vi "cm2nm_find_pairs_of_fiducials.vi"(3 "CurrentSessionFiducialLocations":cluster{"X":dbl, "Y":dbl, "Z":dbl}[](array[cluster]), 4 "ReferenceFiducialLocations":cluster{"X":dbl, "Y":dbl, "Z":dbl}[](array[cluster])) -> (0 "IndexRefrenceSession":i32[](array[numeric]), 1 "min_distance":dbl, 2 "IndexCurrentSession":i32[](array[numeric]))   [LabVIEW 2011]
doc: "from two sessions resolve the pairing of the fiducials from the location. assumes the session with the least number of fiducials is a subset of the equal or larger set of fiducials."
panel:
  in  "index":i32
  in  "stop":bool
  out "XY Graph":cluster{dbl[], dbl[]}[](graph)
  out "Waveform Graph":dbl[](graph)
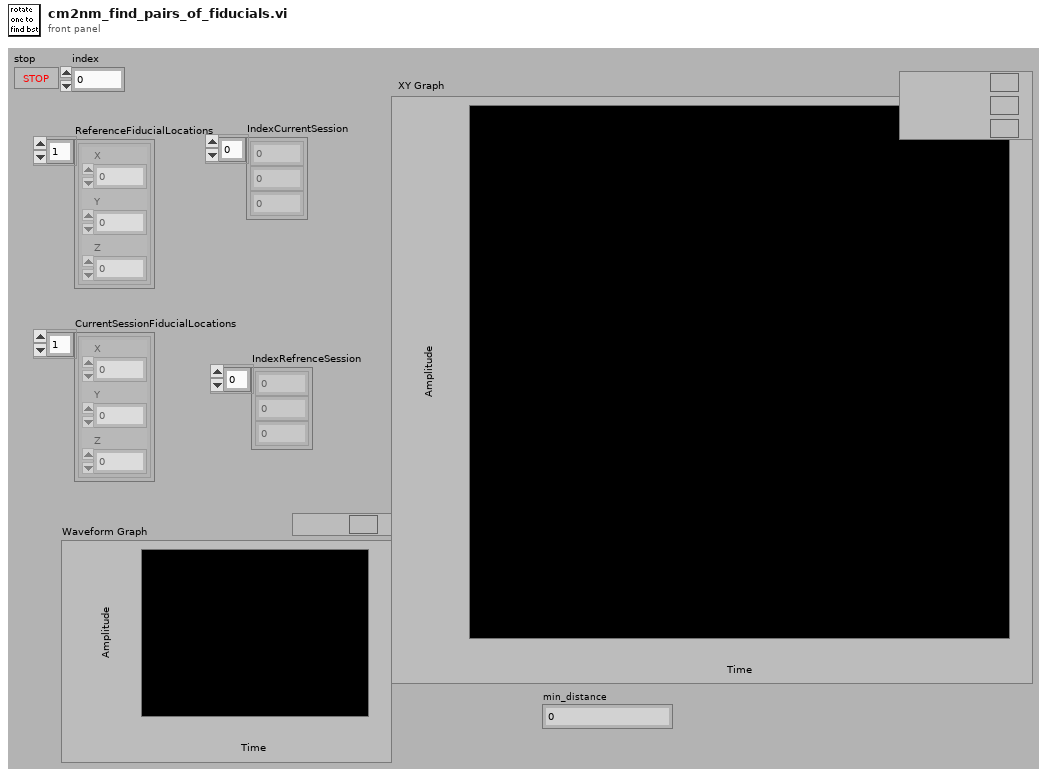
[diagram p1: front panel]
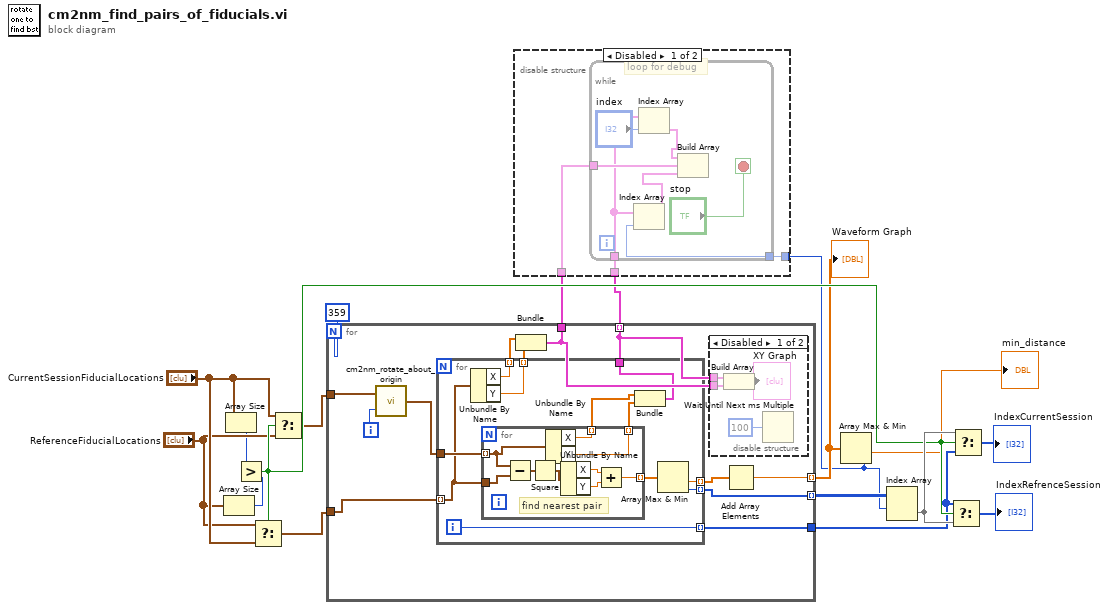
[diagram p0: block diagram]
diagram:
  n1 = Array Size(array="ReferenceFiducialLocations") -> (size(s)=w8:i32)
  n2 = Array Size(array="CurrentSessionFiducialLocations") -> (size(s)=w7:i32)
  n3 = Greater?(x=w7, y=w8) -> (0:w14:bool)
  n4 = Select(t="ReferenceFiducialLocations", s=w14, f="CurrentSessionFiducialLocations") -> (s? t:f=w13:cluster{"X":dbl, "Y":dbl, "Z":dbl}[])
  n5 = Select(t="CurrentSessionFiducialLocations", s=w14, f="ReferenceFiducialLocations") -> (s? t:f=w11:cluster{"X":dbl, "Y":dbl, "Z":dbl}[])
  n6 = for {
    N: 359 -> [_]
    tunnel: w11 -> [w30]
    tunnel: w13 -> [w24]
    tunnel: [w28] -> w10 mode=indexing
    tunnel: [w27] -> w9 mode=indexing
    tunnel: [w26] -> w5
    tunnel: [w19] -> w4
    tunnel: [w20] -> w3 mode=indexing
    i -> [w23]
    n7 = call "cm2nm_rotate_about_origin.vi"("Theta(deg)"=w23, "In"=w30) -> ("Rotated"=w25:cluster{"X":dbl, "Y":dbl, "Z":dbl}[])
    n8 = for {
      tunnel: w24 -> [w40] mode=indexing
      tunnel: w25 -> [w45]
      tunnel: [w43] -> w29 mode=indexing
      tunnel: [w42] -> w28 mode=indexing
      tunnel: [w41] -> w26 mode=indexing
      tunnel: [w37] -> w20
      tunnel: [w36] -> w22 mode=indexing
      tunnel: [w35] -> w21 mode=indexing
      i -> [w41]
      n9 = Unbundle By Name(w40) -> ("X"=w36:dbl, "Y"=w35:dbl)
      n10 = for {
        tunnel: w45 -> [w49] mode=indexing
        tunnel: w40 -> [w54]
        tunnel: [w51] -> w44 mode=indexing
        tunnel: [w47] -> w39 mode=indexing
        tunnel: [w46] -> w38 mode=indexing
        # "find nearest pair"
        n11 = Subtract(x=w49, y=w54) -> (x-y=w50:cluster{"X":dbl, "Y":dbl, "Z":dbl})
        n12 = Square(x=w50) -> (x^2=w53:cluster{"X":dbl, "Y":dbl, "Z":dbl})
        n13 = Unbundle By Name(w49) -> ("X"=w47:dbl, "Y"=w46:dbl)
        n14 = Unbundle By Name(w53) -> ("X"=w48:dbl, "Y"=w52:dbl)
        n15 = Add(x=w48, y=w52) -> (x+y=w51:dbl)
      }
      n16 = Bundle(w39, w38) -> (w37:cluster{dbl[], dbl[]})  [unwired: 1 out]
      n17 = Array Max & Min(array=w44) -> (min value=w43:dbl, min index (indices)=w42:i32)  [unwired: 2 out]
    }
    n18 = Bundle(w22, w21) -> (w19:cluster{dbl[], dbl[]})  [unwired: 1 out]
    n19 = disable-structure shown="Disabled" {
      disable-tunnel: w20 -> [w34 _]
      disable-tunnel: w19 -> [w33 _]
      frame Disabled {
        n20 = Build Array(w34, w33) -> (→"XY Graph":cluster{dbl[], dbl[]}[])
        n21 = Wait Until Next ms Multiple(millisecond multiple=u32 100) -> ()  [unwired: 1 out]
      }
      frame Enabled {
      }
    }
    n22 = Add Array Elements(numeric array=w29) -> (sum=w27:dbl)
  }
  "Waveform Graph" <- w9
  n23 = Array Max & Min(array=w9) -> (min value=→"min_distance":dbl, min index (indices)=w2:i32)  [unwired: 2 out]
  n24 = disable-structure shown="Disabled" {
    disable-tunnel: w4 -> [w57 _]
    disable-tunnel: w3 -> [w56 _]
    disable-tunnel: w2 -> [w55 _]
    frame Disabled {
      # "loop for debug"
      n25 = while {
        tunnel: w57 -> [w65]
        tunnel: w56 -> [w60]
        tunnel: w55 -> [w63]
        stop <- "stop" stop-if-true
        n26 = Index Array(array=w60, index=w63) -> (element=w62:cluster{dbl[], dbl[]})
        n27 = Index Array(array=w60, index="index") -> (element=w58:cluster{dbl[], dbl[]})
        n28 = Build Array(w58, w65, w62) -> (w64:cluster{dbl[], dbl[]}[])
      }
    }
    frame Enabled {
    }
  }
  n29 = Index Array(array=w10, index (row)=w2) -> (element=w16:i32[])  [unwired: 1 in]
  n30 = Select(t=w5, s=w14, f=w16) -> (s? t:f=→"IndexRefrenceSession":i32[])
  n31 = Select(t=w16, s=w14, f=w5) -> (s? t:f=→"IndexCurrentSession":i32[])
